vi "IsLatching.vi"(8 "error in":errorcluster, 11 "Control Terminal in":refnum<class "ControlTerminal.lvclass">) -> (0 "error out":errorcluster, 2 "latching":bool, 3 "Control Terminal out":refnum<class "ControlTerminal.lvclass">)   [LabVIEW 2014, in "ControlTerminal.lvclass"]
uses:
  ControlTerminal.lvclass
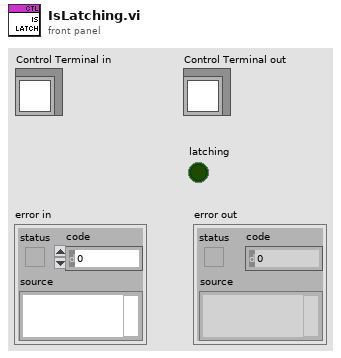
[diagram p1: front panel]
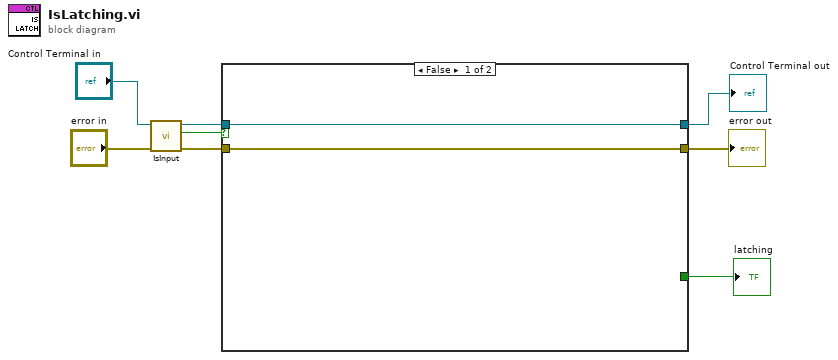
[diagram p0: block diagram]
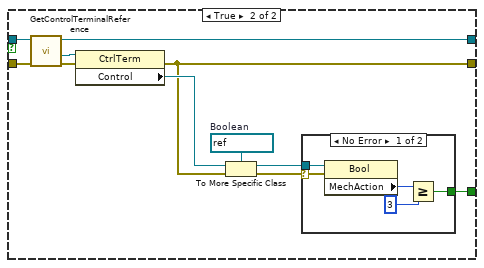
[diagram p2: hidden frame]
diagram:
  n1 = call-dynamic "IsInput.vi"("error in"="error in", "ControlTerminal in"="Control Terminal in") -> ("error out"=w2:errorcluster, "input"=w4:bool, "ControlTerminal out"=w5:refnum<class "ControlTerminal.lvclass">)  [unwired: 5 in]
  n2 = case shown="False" w4 {
    tunnel: w2 -> [w10 w13]
    tunnel: [w10 w20] -> w8
    tunnel: [_ w16] -> w7
    tunnel: w5 -> [w9 w12]
    tunnel: [w9 w11] -> w1
    frame False {
    }
    frame True {
      w19 = refnum<vi> refnum  # Boolean
      n3 = call "GetControlTerminalReference.vi"("error in"=w13, "ControlTerminal in"=w12) -> ("error out"=w14:errorcluster, "reference"=w15:refnum<vi>, "ControlTerminal out"=w11:refnum<class "ControlTerminal.lvclass">)  [unwired: 7 in]
      n4 = property class="CtrlTerm"(reference=w15, error in=w14) -> (error out=w20:errorcluster, "Control"=w21:refnum<vi>)  [unwired: 1 out]
      n5 = To More Specific Class(target class=w19, reference=w21, error in=w20) -> (specific class reference=w17:refnum<vi>, error out=w18:errorcluster)
      n6 = case shown="No Error" w18 {
        selector: w18 -> [w26 _]
        tunnel: w17 -> [w25 _]
        tunnel: [w22 _] -> w16
        frame No Error {
          n7 = property class="Bool"(reference=w25, error in=w26) -> ("MechAction"=w24:u32)  [unwired: 2 out]
          n8 = Greater Or Equal?(x=w24, y=u32 3) -> (x >= y?=w22:bool)
        }
        frame Error {
        }
      }
    }
  }
  "error out" <- w8
  "Control Terminal out" <- w1
  "latching" <- w7
